vi "JAUS ComplexServices.vi"() -> ()   [LabVIEW 2009]
uses:
  Support Files/Complex Services Statechart/Complex Services Queue Element.ctl
  Support Files/Complex Services Statechart/ComplexServices.lvsc/Trigger.ctl
  Support Files/Address.ctl
  Support Files/JUDP Write Queue Element.ctl
  cRIO/Functional Global Variables/Actions for FG's.ctl
  Support Files/Complex Services Statechart/ComplexServices.lvsc/Inputs.ctl
  <vilib>/Statechart/Infrastructure/RTStatechart/RunTime SCN.xnode
  Support Files/Complex Services Statechart/ComplexServices.lvsc
  Support Files/Complex Services Statechart/ComplexServices.lvsc/CompanionDiagram.vi/28/SC Main.vi
  Support Files/Complex Services Statechart/ComplexServices.lvsc/CompanionDiagram.vi
  <vilib>/Statechart/Common/IntGuid.ctl
  <vilib>/Statechart/Common/DbgID.ctl
  Support Files/ServiceRec.ctl
  Support Files/Complex Services Statechart/ComplexServices.lvsc/Outputs.ctl
  <vilib>/Statechart/Common/NI_SC_LVSCCommonFiles.lvlib
panel:
  out "Local Pose Sensor Added?":bool
  out "Local Waypoint List Driver Added?":bool
  out "List Manager Added?":bool
  out "Access Control Added?":bool
  out "HB":bool
  out "Management Added?":bool
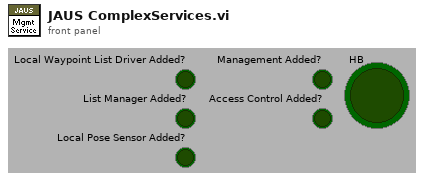
[diagram p1: front panel]
types:
  T1 = typedef "Actions for FG's.ctl" = enum16{"Read", "Write"}
  T2 = typedef "JUDP Write Queue Element.ctl" = cluster{"Encoded JAUS Message":string, "Destination ID":u32}
  T3 = typedef "Complex Services Queue Element.ctl" = cluster{"Trigger":T4, "Payload":string, "Sender ID":T5}
  T4 = typedef "ComplexServices.lvsc/Trigger.ctl" = enum16{"NULL", "ReceiveRequestControl", "ReceiveQueryControl", "ReceiveShutdown", "ReceiveQueryStatus", "ReceiveStandby", "ReceiveResume", "Timeout", "Initialized", "Failure", "ReceiveQueryLocalPose", "ReceiveSetLocalPose", "ReceiveQueryElementList", "ReceiveQueryElementCount", "ReceiveSetElement", "ReceiveExecuteList", "ReceiveQueryTravelSpeed", "ReceiveQueryLocalWaypoint", "ReceiveQueryActiveElement"}
  T5 = typedef "Address.ctl" = cluster{"Subsystem Id":u16, "Node Id":u8, "Component Id":u8}
  T6 = typedef "ServiceRec.ctl" = cluster{"ServiceURI":string, "MajorVerNum":u8, "MinorVerNum":u8}
  T7 = typedef "NI_SC_LVSCCommonFiles.lvlib/IntGuid.ctl" = cluster{"Data1":u32, "Data2":u16, "Data3":u16, "Data4":u8, "Data5":u8, "Data6":u8, "Data11":u8, "Data9":u8, "Data10":u8, "Data8":u8, "Data7":u8}
  T8 = typedef "NI_SC_LVSCCommonFiles.lvlib/DbgID.ctl" = cluster{"VIRef":u32, "IntGUID":T7}
  T9 = typedef "ComplexServices.lvsc/Inputs.ctl" = cluster{"Payload":string, "Sender ID":T5, "JUDP Write Queue ref":refnum<queue>}
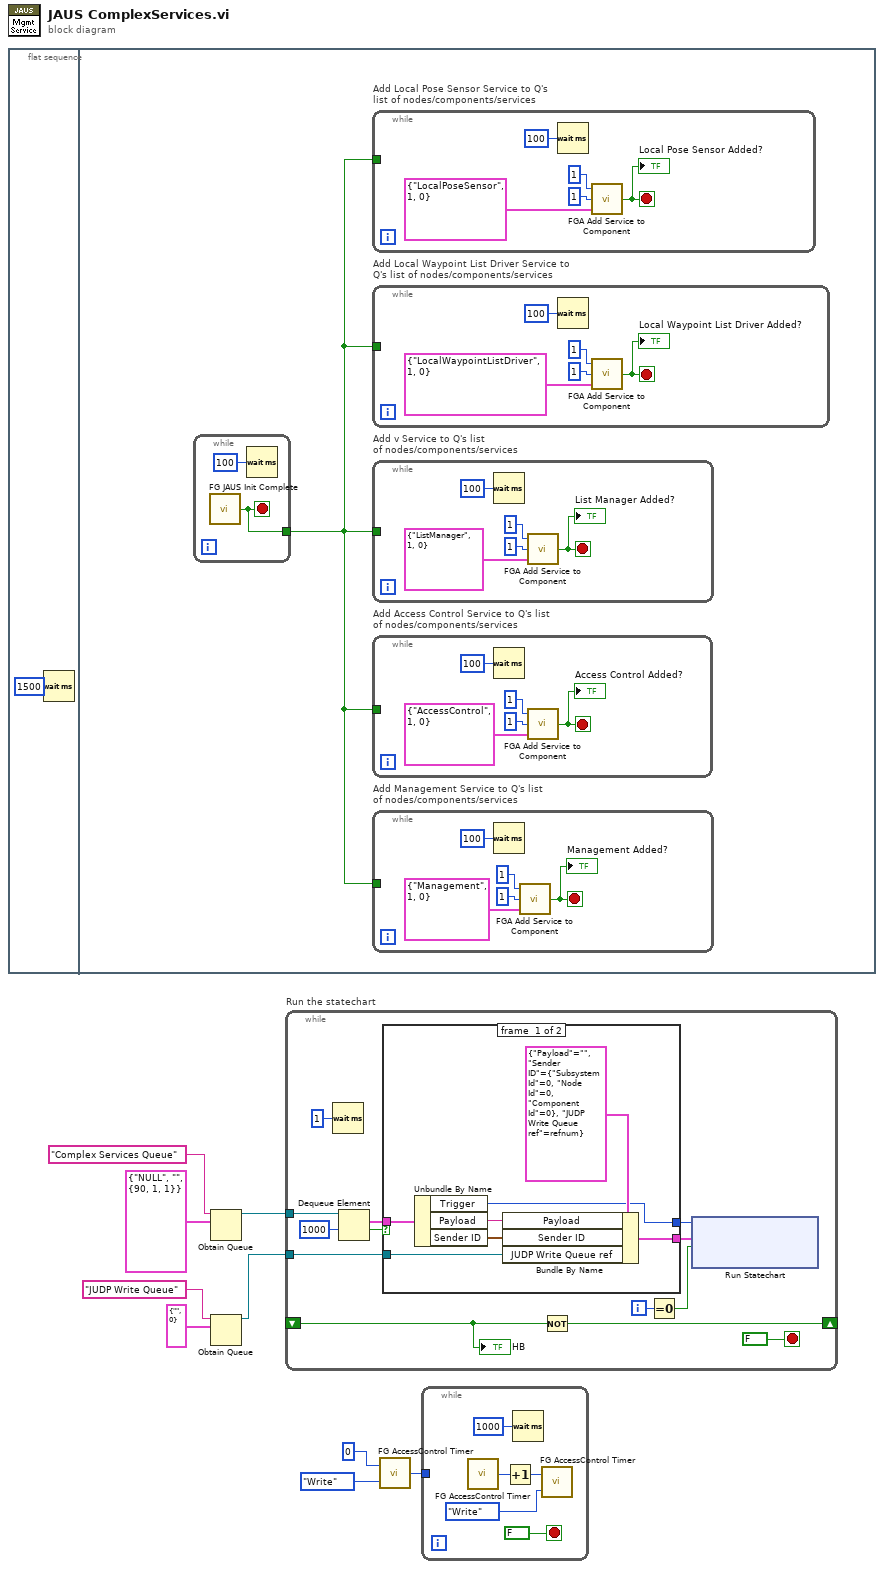
[diagram p0: block diagram]
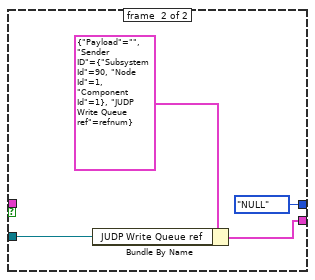
[diagram p2: hidden frame]
diagram:
  n1 = flat-sequence {
    frame #0 {
      n2 = Wait (ms)(milliseconds to wait=u32 1500) -> ()  [unwired: 1 out]
    }
    frame #1 {
      n3 = while "sdvsd" {
        tunnel: [w12] -> w11
        stop <- w12 stop-if-true
        n4 = call "FG JAUS Init Complete.vi"() -> ("Init Complete out"=w12:bool)  [unwired: 2 in]
        n5 = Wait (ms)(milliseconds to wait=u32 100) -> ()  [unwired: 1 out]
      }
      n6 = while "Add Local Pose Sensor Service to Q's \nlist of nodes/components/services" {
        tunnel: w11 -> [_]
        stop <- w15 stop-if-true
        n7 = Wait (ms)(milliseconds to wait=u32 100) -> ()  [unwired: 1 out]
        n8 = call "FGA Add Service to Component.vi"("ServiceRec"=T6 {"ServiceURI"="LocalPoseSensor", "MajorVerNum"=1, "MinorVerNum"=0}, "Component Id"=u8 1, "Node Id"=u8 1) -> ("Added?"=w15:bool)
        "Local Pose Sensor Added?" <- w15
      }
      n9 = while "Add Local Waypoint List Driver Service to \nQ's list of nodes/components/services" {
        tunnel: w11 -> [_]
        stop <- w20 stop-if-true
        n10 = Wait (ms)(milliseconds to wait=u32 100) -> ()  [unwired: 1 out]
        n11 = call "FGA Add Service to Component.vi"("ServiceRec"=T6 {"ServiceURI"="LocalWaypointListDriver", "MajorVerNum"=1, "MinorVerNum"=0}, "Component Id"=u8 1, "Node Id"=u8 1) -> ("Added?"=w20:bool)
        "Local Waypoint List Driver Added?" <- w20
      }
      n12 = while "Add v Service to Q's list \nof nodes/components/services" {
        tunnel: w11 -> [_]
        stop <- w25 stop-if-true
        n13 = Wait (ms)(milliseconds to wait=u32 100) -> ()  [unwired: 1 out]
        n14 = call "FGA Add Service to Component.vi"("ServiceRec"=T6 {"ServiceURI"="ListManager", "MajorVerNum"=1, "MinorVerNum"=0}, "Component Id"=u8 1, "Node Id"=u8 1) -> ("Added?"=w25:bool)
        "List Manager Added?" <- w25
      }
      n15 = while "Add Access Control Service to Q's list \nof nodes/components/services" {
        tunnel: w11 -> [_]
        stop <- w30 stop-if-true
        n16 = Wait (ms)(milliseconds to wait=u32 100) -> ()  [unwired: 1 out]
        n17 = call "FGA Add Service to Component.vi"("ServiceRec"=T6 {"ServiceURI"="AccessControl", "MajorVerNum"=1, "MinorVerNum"=0}, "Component Id"=u8 1, "Node Id"=u8 1) -> ("Added?"=w30:bool)
        "Access Control Added?" <- w30
      }
      n18 = while "Add Management Service to Q's list \nof nodes/components/services" {
        tunnel: w11 -> [_]
        stop <- w35 stop-if-true
        n19 = Wait (ms)(milliseconds to wait=u32 100) -> ()  [unwired: 1 out]
        n20 = call "FGA Add Service to Component.vi"("ServiceRec"=T6 {"ServiceURI"="Management", "MajorVerNum"=1, "MinorVerNum"=0}, "Component Id"=u8 1, "Node Id"=u8 1) -> ("Added?"=w35:bool)
        "Management Added?" <- w35
      }
    }
  }
  n21 = Obtain Queue(name (unnamed)="Complex Services Queue", element data type=T3 {"Trigger"=enum."NULL", "Payload"="", "Sender ID"={"Subsystem Id"=90, "Node Id"=1, "Component Id"=1}} ("Receive FSM Queue Element")) -> (queue out=w8:refnum<queue>)  [unwired: 3 in, 2 out]
  n22 = Obtain Queue(name (unnamed)="JUDP Write Queue", element data type=T2 {"Encoded JAUS Message"="", "Destination ID"=0} ("JUDP Send Queue Element")) -> (queue out=w4:refnum<queue>)  [unwired: 3 in, 2 out]
  n23 = while "Run the statechart" {
    tunnel: w8 -> [w51]
    tunnel: w4 -> [w47]
    shift-right: [w44] -> _
    shift-left: _ -> [w45]
    i -> [w39]
    stop <- FALSE stop-if-true
    n24 = Wait (ms)(milliseconds to wait=u32 1) -> ()  [unwired: 1 out]
    n25 = Dequeue Element(queue=w51, timeout in ms (-1)=1000) -> (element=w49:T3, timed out?=w48:bool)  [unwired: 1 in, 2 out]
    n26 = case shown="True" w48 {
      tunnel: w49 -> [w74 _]
      tunnel: w47 -> [w71 w77]
      tunnel: [w70 Trigger."NULL" ("Trigger")] -> w42
      tunnel: [w69 w78] -> w41
      frame #0 {
        n27 = Unbundle By Name(w74) -> ("Trigger"=w70:T4, "Payload"=w72:string, "Sender ID"=w73:T5)
        n28 = Bundle By Name(cluster=T9 {"Payload"="", "Sender ID"={"Subsystem Id"=0, "Node Id"=0, "Component Id"=0}, "JUDP Write Queue ref"=refnum} ("Inputs"), "Payload"=w72, "Sender ID"=w73, "JUDP Write Queue ref"=w71) -> (w69:T9)
      }
      frame #1 {
        n29 = Bundle By Name(cluster=T9 {"Payload"="", "Sender ID"={"Subsystem Id"=90, "Node Id"=1, "Component Id"=1}, "JUDP Write Queue ref"=refnum} ("Inputs"), "JUDP Write Queue ref"=w77) -> (w78:T9)
      }
    }
    n30 = Not(x=w45) -> (.not. x?=w44:bool)
    n31 = Equal To 0?(x=w39) -> (x = 0?=w40:bool)
    n32 = xnode "Run Statechart"("Init?"=w40, "Inputs"=w41, "Trigger"=w42) -> ()  [unwired: 2 out]
    "HB" <- w45
  }
  n33 = call "FG AccessControl Timer.vi"("FG Action (Read)"=Actions_for_FG's."Write", "Count in"=0) -> ("Count out"=w3:i32)
  n34 = while {
    tunnel: w3 -> [_]
    stop <- FALSE stop-if-true
    n35 = call "FG AccessControl Timer.vi"() -> ("Count out"=w82:i32)  [unwired: 2 in]
    n36 = Increment(x=w82) -> (x+1=w81:i32)
    n37 = Wait (ms)(milliseconds to wait=u32 1000) -> ()  [unwired: 1 out]
    n38 = call "FG AccessControl Timer.vi"("FG Action (Read)"=Actions_for_FG's."Write", "Count in"=w81) -> ()  [unwired: 1 out]
  }
